vi "SpecAn Setup.vi"(0 "VISA In":refnum<visa-resource-name>, 1 "SpecAn Cluster":T1={"Span (Hz)"=0.0, "Center Freq (Hz)"=0.0, "Mode"=0, "Frequency Ref In"=0, "Trace Type"=0, "Trace"=1, "Enable Trace Update"=FALSE, "Enable Trace Display"=FALSE, "Manual VBW"=3000001, "Auto VBW"=TRUE, "Manual RBW"=3000000, "Auto RBW"=TRUE, "Amplitude Units"=0, "Reference Level"=0.0, "Reference Level Offset"=0.0, "Averaging On/Off"=0, "Marker Type"=0, "Readout"=0, "Active Marker"=1, "Auto Align Enable"=enum."Disable"} {"Active Marker" items=["Marker1"=1, "Marker2"=2, "Marker3"=3, "Marker4"=4, "Marker5"=5, "Marker6"=6, "Marker7"=7, "Marker8"=8, "Marker9"=9, "Marker10"=10, "Marker11"=11, "Marker12"=12]; "Readout" items=["Auto", "Frequency", "Period", "Time", "Inverse Time"]; "Marker Type" items=["Normal", "Delta", "Fixed", "Off"]; "Averaging On/Off" items=["OFF", "ON"]; "Amplitude Units" items=["dBm", "dBmV", "dBmA", "W", "V", "A", "dBuV", "dBuA"]; "Manual RBW" format="%#.5p"; "Manual VBW" format="%#.5p"; "Trace" items=["Trace 1"=1, "Trace 2"=2, "Trace 3"=3, "Trace 4"=4, "Trace 5"=5, "Trace 6"=6]; "Trace Type" items=["Clear Write", "Average", "Maximum Hold", "Minimum Hold"]; "Frequency Ref In" items=["Internal", "External"]; "Mode" items=["Swept SA", "Channel Power", "Occupied Bandwidth", "Power Stat CCDF", "Adjacent Channel Power", "Burst Power", "Spurious Emissions", "Spectrum Emission Mask", "List Sweep", "TOI", "Harmonic"]; "Center Freq (Hz)" format="%#_6p"; "Span (Hz)" format="%#_6p"}, 5 "Error In":errorcluster) -> (14 "VISA Out":refnum<visa-resource-name>, 19 "Error Out":errorcluster)   [LabVIEW 2015]
uses:
  Controls/SpecAn Cluster.ctl
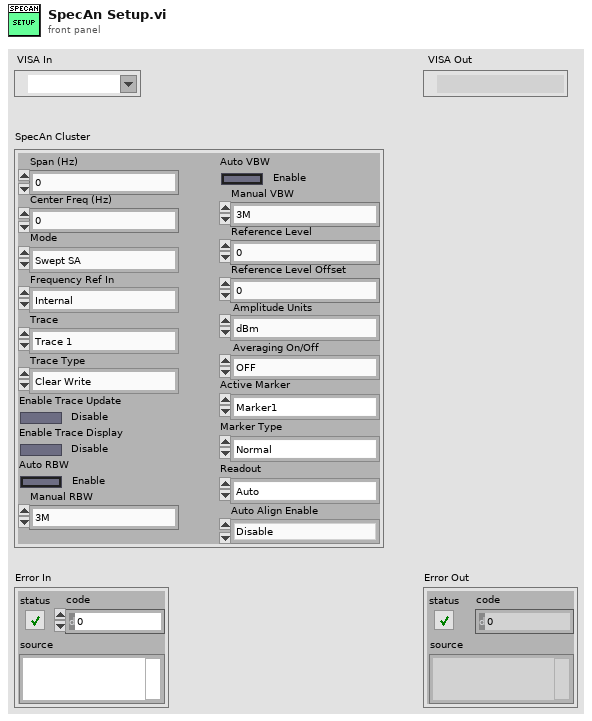
[diagram p1: front panel]
types:
  T1 = typedef "SpecAn Cluster.ctl" = cluster{"Span (Hz)":dbl, "Center Freq (Hz)":dbl, "Mode":i32, "Frequency Ref In":i32, "Trace Type":i32, "Trace":i32, "Enable Trace Update":bool, "Enable Trace Display":bool, "Manual VBW":i32, "Auto VBW":bool, "Manual RBW":i32, "Auto RBW":bool, "Amplitude Units":i32, "Reference Level":dbl, "Reference Level Offset":dbl, "Averaging On/Off":i32, "Marker Type":i32, "Readout":i32, "Active Marker":i32, "Auto Align Enable":enum16{"Disable", "Enable"}}
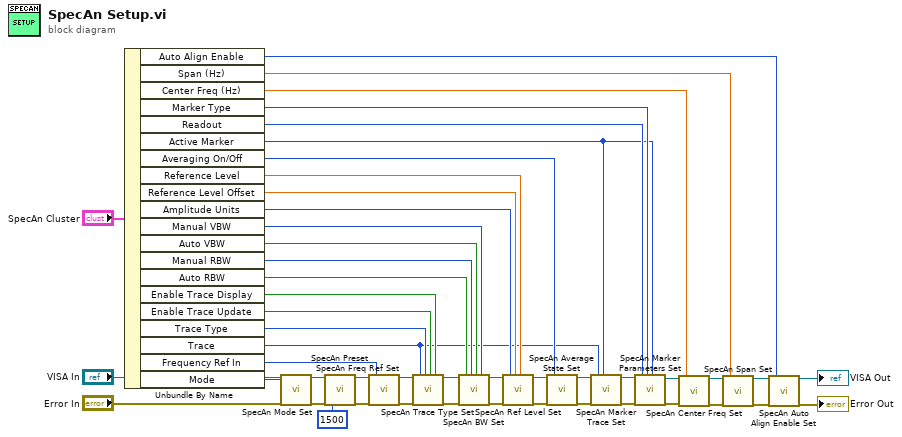
[diagram p0: block diagram]
diagram:
  n1 = Unbundle By Name("SpecAn Cluster") -> ("Auto Align Enable"=w12:enum16{"Disable", "Enable"}, "Span (Hz)"=w15:dbl, "Center Freq (Hz)"=w16:dbl, "Marker Type"=w23:i32, "Readout"=w24:i32, "Active Marker"=w22:i32, "Averaging On/Off"=w26:i32, "Reference Level"=w28:dbl, "Reference Level Offset"=w29:dbl, "Amplitude Units"=w30:i32, "Manual VBW"=w31:i32, "Auto VBW"=w32:bool, "Manual RBW"=w33:i32, "Auto RBW"=w34:bool, "Enable Trace Display"=w35:bool, "Enable Trace Update"=w36:bool, "Trace Type"=w37:i32, "Trace"=w25:i32, "Frequency Ref In"=w38:i32, "Mode"=w39:i32)
  n2 = call "SpecAn Mode Set.vi"("VISA In"="VISA In", "Error In"="Error In", "Mode (0: Swept SA)"=w39) -> ("VISA Out"=w9:refnum<visa-resource-name>, "Error Out"=w8:errorcluster)  [unwired: 15 in]
  n3 = call "SpecAn Preset.vi"("VISA In"=w9, "Error In"=w8, "Delay (ms)"=u32 1500) -> ("VISA Out"=w10:refnum<visa-resource-name>, "Error Out"=w11:errorcluster)  [unwired: 15 in]
  n4 = call "SpecAn Freq Ref Set.vi"("VISA In"=w10, "Error In"=w11, "Freq Ref"=w38) -> ("VISA Out"=w43:refnum<visa-resource-name>, "Error Out"=w44:errorcluster)  [unwired: 15 in]
  n5 = call "SpecAn Trace Type Set.vi"("VISA In"=w43, "Error In"=w44, "Trace"=w25, "Trace Type"=w37, "Enable Trace Update (F: Disable)"=w36, "Enable Trace Display (F: Disable)"=w35) -> ("VISA Out"=w3:refnum<visa-resource-name>, "Error Out"=w6:errorcluster)  [unwired: 12 in]
  n6 = call "SpecAn BW Set.vi"("VISA In"=w3, "Error In"=w6, "Auto RBW (T: Enable)"=w34, "Manual RBW"=w33, "Auto VBW (T: Enable)"=w32, "Manual VBW"=w31) -> ("VISA Out"=w2:refnum<visa-resource-name>, "Error Out"=w41:errorcluster)  [unwired: 12 in]
  n7 = call "SpecAn Ref Level Set.vi"("VISA In"=w2, "Error In"=w41, "Amplitude Units (0: dBm)"=w30, "Reference Level Offset (0 dB)"=w29, "Reference Level (0 dBm)"=w28) -> ("VISA Out"=w40:refnum<visa-resource-name>, "Error Out"=w42:errorcluster)  [unwired: 13 in]
  n8 = call "SpecAn Average State Set.vi"("VISA In"=w40, "Error In"=w42, "Averaging On/Off"=w26) -> ("VISA Out"=w27:refnum<visa-resource-name>, "Error Out"=w19:errorcluster)  [unwired: 15 in]
  n9 = call "SpecAn Marker Trace Set.vi"("VISA In"=w27, "Error In"=w19, "Marker Trace"=w25, "Active Marker"=w22) -> ("VISA Out"=w21:refnum<visa-resource-name>, "Error Out"=w20:errorcluster)  [unwired: 14 in]
  n10 = call "SpecAn Marker Parameters Set.vi"("VISA In"=w21, "Error In"=w20, "Readout"=w24, "Marker Type"=w23, "Active Marker"=w22) -> ("VISA Out"=w18:refnum<visa-resource-name>, "Error Out"=w17:errorcluster)  [unwired: 13 in]
  n11 = call "SpecAn Center Freq Set.vi"("VISA In"=w18, "Error In"=w17, "Center Freq (Hz)"=w16) -> ("VISA Out"=w48:refnum<visa-resource-name>, "Error Out"=w47:errorcluster)  [unwired: 15 in]
  n12 = call "SpecAn Span Set.vi"("VISA In"=w48, "Error In"=w47, "Span (Hz)"=w15) -> ("VISA Out"=w4:refnum<visa-resource-name>, "Error Out"=w5:errorcluster)  [unwired: 15 in]
  n13 = call "SpecAn Auto Align Enable Set.vi"("VISA In"=w4, "Error In"=w5, "Auto Align Enable"=w12) -> ("VISA Out"=→"VISA Out":refnum<visa-resource-name>, "Error Out"=→"Error Out":errorcluster)  [unwired: 15 in]
